vi "2 DirectionChangeGoodness.vi"(1 "Test Heading":dbl=57.0) -> (0 "Goodness":dbl=0.027051846866350416)   [LabVIEW 2011]
doc: "The DirectionChangeGoodness VI outputs a value between 1 and 0 that represents the goodness of the hypothetical heading from the perspective of turning as little as possible."
uses:
  2 Typedefs/heading.ctl
  2 Globals/2 Global.vi
  2 Globals/2 TuningConstants.vi
panel:
  out "Wind Adjustment":dbl=0.2
  in  "Tuning Quotient":i32=240
  out "Current Heading":T1 format="%05.1f"
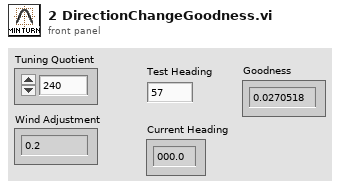
[diagram p1: front panel]
types:
  T1 = typedef "heading.ctl" = dbl
  T2 = typedef "apparent wind.ctl" = cluster{"Toward Fore":dbl, "Toward Starboard":dbl}
  T3 = typedef "robot velocity.ctl" = cluster{"East":dbl, "North":dbl}
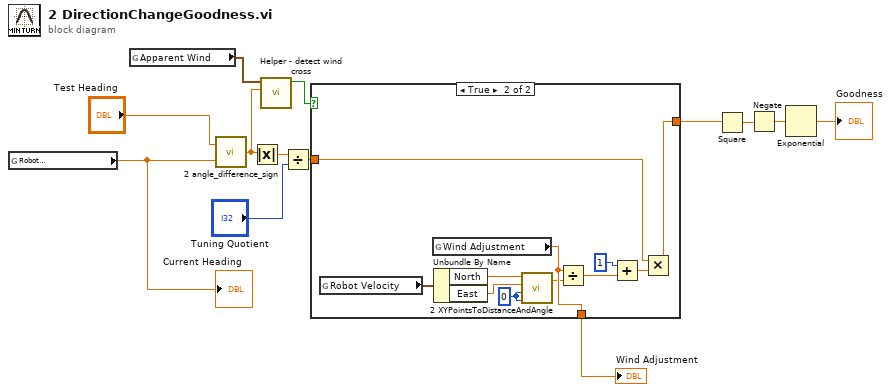
[diagram p0: block diagram]
diagram:
  n1 = global read "2 Global.vi" "Robot\nHeading"() -> (w9:T1)
  "Current Heading" <- w9
  n2 = global read "2 Global.vi" "Apparent Wind"() -> (w5:T2)
  n3 = call "2 angle_difference_sign.vi"("Angle 2"=w9, "Angle 1"="Test Heading") -> ("Difference"=w2:dbl)
  n4 = Absolute Value(x=w2) -> (abs(x)=w4:dbl)
  n5 = call "Helper - detect wind cross.vi"("Heading Change"=w2, "Apparent Wind"=w5) -> ("Crossing Wind?"=w3:bool)  [unwired: 9 in]
  n6 = Divide(x=w4, y="Tuning Quotient") -> (x/y=w7:dbl)
  n7 = case shown="True" w3 {
    tunnel: [w14 w24] -> w6
    tunnel: w7 -> [w14 w25]
    tunnel: [_ w17] -> w1
    frame False {
    }
    frame True {
      w21 = 0
      n8 = global read "2 Global.vi" "Robot Velocity"() -> (w18:T3)
      n9 = global read "2 TuningConstants.vi" "Wind Adjustment"() -> (w17:dbl)
      n10 = Unbundle By Name(w18) -> ("North"=w20:dbl, "East"=w19:dbl)
      n11 = call "2 XYPointsToDistanceAndAngle.vi"("East 2"=w21, "North 2"=w21, "East 1"=w19, "North 1"=w20) -> ("Distance"=w16:dbl)  [unwired: 1 out]
      n12 = Divide(x=w17, y=w16) -> (x/y=w15:dbl)
      n13 = Add(x=1, y=w15) -> (x+y=w22:dbl)
      n14 = Multiply(x=w25, y=w22) -> (x*y=w24:dbl)
    }
  }
  "Wind Adjustment" <- w1
  n15 = Square(x=w6) -> (x^2=w11:dbl)
  n16 = Negate(x=w11) -> (-x=w12:dbl)
  n17 = Exponential(1:w12) -> (0:→"Goodness":dbl)
